vi "Get Triggered Block.vi"(6 "Bytes per sample":i32, 7 "Samples per trigger increment":i32=2, 8 "error in (no error)":errorcluster, 9 "Post-trigger samples":u64=11534336 format="0x%x (%d)", 10 "Pre-trigger samples":i32=-100000 format="0x%x (%d)", 11 "RP Communicator in":refnum<class "RP Communicator.lvclass">) -> (0 "error out":errorcluster, 2 "data out":string, 3 "RP Communicator out":refnum<class "RP Communicator.lvclass">)   [LabVIEW 2015, in "RP Communicator.lvclass"]
uses:
  RP Communicator.lvclass
  RP Communicator.lvclass/RP Communicator.ctl
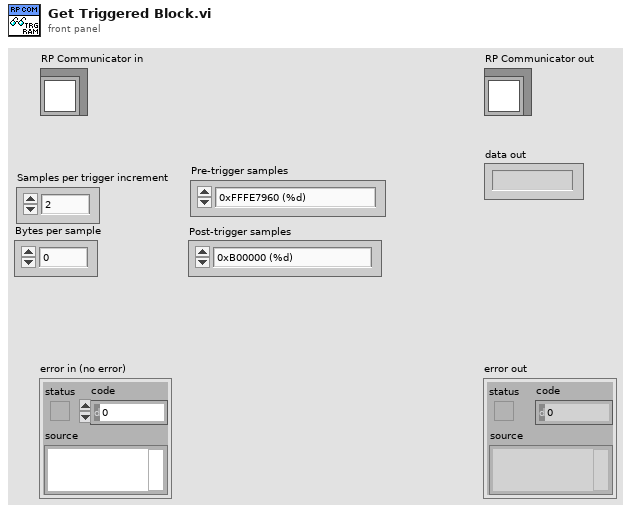
[diagram p1: front panel]
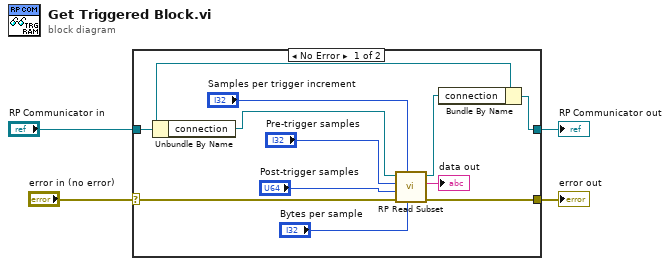
[diagram p0: block diagram]
diagram:
  n1 = case shown="No Error" "error in (no error)" {
    selector: "error in (no error)" -> [w7 w17]
    tunnel: [w10 w17] -> w3
    tunnel: [w14 w16] -> w1
    tunnel: "RP Communicator in" -> [w15 w16]
    frame No Error {
      n2 = Unbundle By Name(w15) -> ("connection"=w13:refnum<k5>)
      n3 = call "RP Read Subset.vi"("Bytes per sample"="Bytes per sample", "Samples per trigger increment"="Samples per trigger increment", "Error In"=w7, "Post-trigger samples"="Post-trigger samples", "Pre-trigger samples"="Pre-trigger samples", "connection ID"=w13) -> ("Error Out"=w10:errorcluster, "Data stream"=→"data out":string, "connection ID out"=w12:refnum<k5>)  [unwired: 2 in, 1 out]
      n4 = Bundle By Name(cluster=w15, "connection"=w12) -> (w14:refnum<class "RP Communicator.lvclass">)
    }
    frame Error {
    }
  }
  "error out" <- w3
  "RP Communicator out" <- w1
